vi "AutoDriver.vi"(0 "NXT In":T4, 1 "Motors":cluster{"TetrixDCMotor":T1, "TetrixDCMotor":T1}, 2 "Direction":T3=enum."Forward", 3 "Speed":T2, 5 "Time (1 sec)":sgl=1.0) -> (6 "NXT Out":T4)   [LabVIEW 2012]
uses:
  <vilib>/NXT/Subs/LVHSConnector.ctl
  <vilib>/NXT/LegoClasses/BrickReference/BrickReference.lvclass
  AutoDriverControl.ctl
  FTC 2012 - 2013/Controls/SpeedControl.ctl
  <vilib>/NXT/Hardware/Plugins/Tetrix DC Motor/TetrixDCMotorAddress.ctl
  <vilib>/NXT/Dual Mode Library/Waits/Wait_Num.vi
  <vilib>/NXT/NXTIO Xnodes/NXTIONodeSubVIs/TETRIX IO Move DC Motors.vi
  <vilib>/NXT/NXTIO Xnodes/NXTIONodeSubVIs/TETRIX IO Stop DC Motors.vi
  <vilib>/NXT/NXTIO Xnodes/NXTIOXNode/NXTIO.xnode
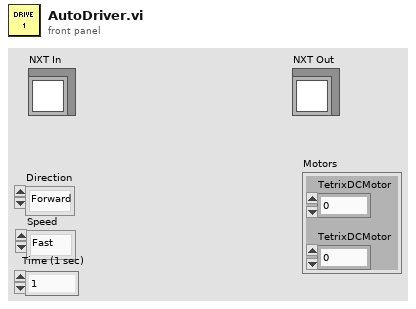
[diagram p1: front panel]
types:
  T1 = typedef "TetrixDCMotorAddress.ctl" = i16
  T2 = typedef "SpeedControl.ctl" = enum16{"Fast", "Medium", "Slow"}
  T3 = typedef "AutoDriverControl.ctl" = enum16{"Init", "Forward", "Reverse", "Left", "Right", "Brake"}
  T4 = typedef "LVHSConnector.ctl" = refnum<class "BrickReference.lvclass">
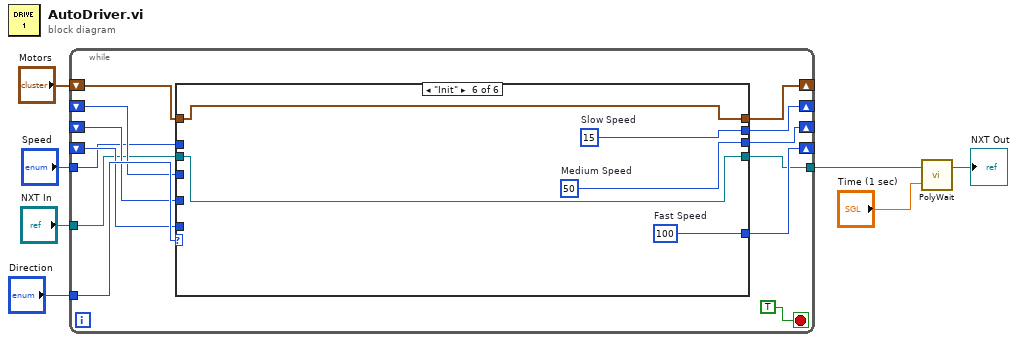
[diagram p0: block diagram]
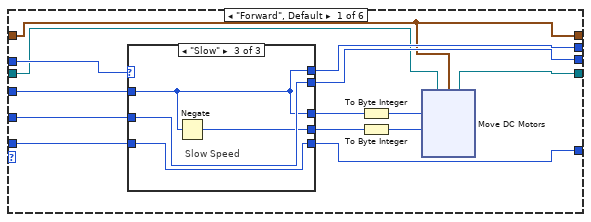
[diagram p2: hidden frame]
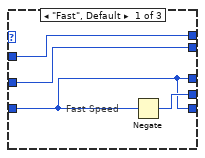
[diagram p3: hidden frame]
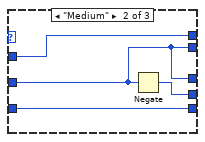
[diagram p4: hidden frame]
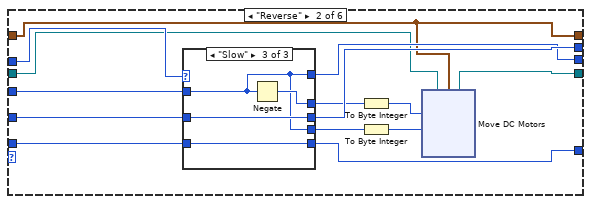
[diagram p5: hidden frame]
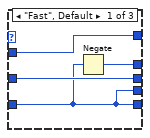
[diagram p6: hidden frame]
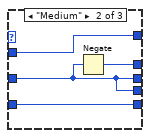
[diagram p7: hidden frame]
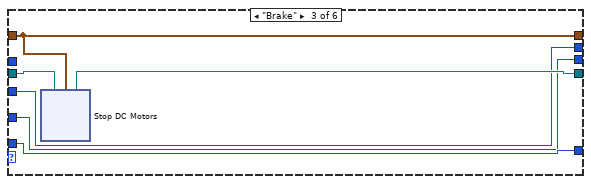
[diagram p8: hidden frame]
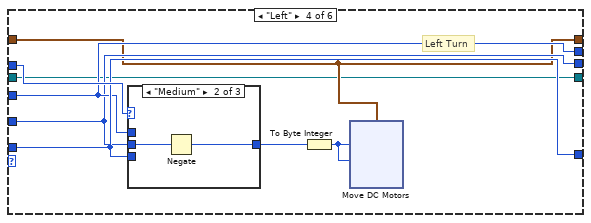
[diagram p9: hidden frame]
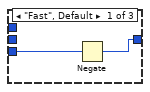
[diagram p10: hidden frame]
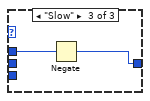
[diagram p11: hidden frame]
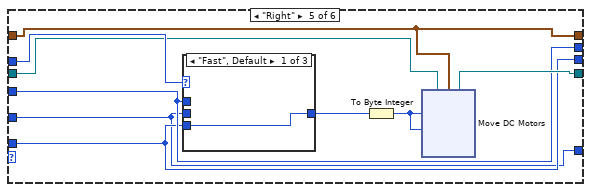
[diagram p12: hidden frame]
diagram:
  n1 = while {
    tunnel: "Direction" -> [w20]
    shift-right: [w10] -> _
    shift-left: _ -> [w17]
    shift-right: [w11] -> _
    shift-left: _ -> [w16]
    shift-right: [w18] -> _
    shift-left: _ -> [w15]
    tunnel: "NXT In" -> [w14]
    tunnel: [w13] -> w4
    tunnel: "Speed" -> [w12]
    shift-right: [w9] -> _
    shift-left: "Motors" -> [w8]
    stop <- TRUE stop-if-true
    n2 = case shown="\"Init\"" w20 {
      tunnel: [w30 w69 w94 w111 w134 w154] -> w10
      tunnel: [w31 w68 w95 w110 w133 w153] -> w11
      tunnel: [w29 w66 w96 w112 w130 w155] -> w18
      tunnel: w17 -> [w34 w63 w94 w111 w134 _]
      tunnel: w16 -> [w33 w62 w95 w110 w130 _]
      tunnel: w15 -> [w32 w70 w96 w112 w133 _]
      tunnel: w14 -> [w27 w65 w98 w108 w136 w156]
      tunnel: [w26 w64 w97 w108 w135 w156] -> w13
      tunnel: w12 -> [w28 w67 _ w113 w138 _]
      tunnel: [w21 w57 w93 w109 w137 w152] -> w9
      tunnel: w8 -> [w21 w57 w93 w109 w137 w152]
      frame "Forward", Default {
        n3 = case shown="\"Slow\"" w28 {
          tunnel: w34 -> [w47 w52 w53]
          tunnel: w33 -> [w48 w49 w55]
          tunnel: w32 -> [w45 w51 w56]
          tunnel: [w48 w49 w55] -> w31
          tunnel: [w47 w52 w53] -> w30
          tunnel: [w45 w51 w56] -> w29
          tunnel: [w46 w50 w54] -> w25
          tunnel: [w45 w49 w53] -> w23
          frame "Fast", Default {
            # "Fast Speed"
            n4 = Negate(x=w45) -> (-x=w46:i32)
          }
          frame "Medium" {
            n5 = Negate(x=w49) -> (-x=w50:i32)
          }
          frame "Slow" {
            # "Slow Speed"
            n6 = Negate(x=w53) -> (-x=w54:i32)
          }
        }
        n7 = To Byte Integer(number=w23) -> (8bit integer=w22:i8)
        n8 = To Byte Integer(number=w25) -> (8bit integer=w24:i8)
        n9 = xnode "Move DC Motors"("Power/Speed 2"=w24, "Power/Speed 1"=w22, "Motors"=w21, "NXT"=w27) -> ("NXT"=w26:T4)
      }
      frame "Reverse" {
        n10 = case shown="\"Slow\"" w67 {
          tunnel: w62 -> [w83 w85 w92]
          tunnel: w63 -> [w84 w88 w89]
          tunnel: w70 -> [w81 w87 w91]
          tunnel: [w84 w88 w89] -> w68
          tunnel: [w83 w85 w92] -> w69
          tunnel: [w82 w86 w90] -> w59
          tunnel: [w81 w87 w91] -> w66
          tunnel: [w81 w85 w89] -> w61
          frame "Fast", Default {
            n11 = Negate(x=w81) -> (-x=w82:i32)
          }
          frame "Medium" {
            n12 = Negate(x=w85) -> (-x=w86:i32)
          }
          frame "Slow" {
            n13 = Negate(x=w89) -> (-x=w90:i32)
          }
        }
        n14 = To Byte Integer(number=w59) -> (8bit integer=w58:i8)
        n15 = To Byte Integer(number=w61) -> (8bit integer=w60:i8)
        n16 = xnode "Move DC Motors"("Power/Speed 2"=w60, "Power/Speed 1"=w58, "Motors"=w57, "NXT"=w65) -> ("NXT"=w64:T4)
      }
      frame "Brake" {
        n17 = xnode "Stop DC Motors"("Motors"=w93, "NXT"=w98) -> ("NXT"=w97:T4)
      }
      frame "Left" {
        # "Left Turn"
        n18 = case shown="\"Medium\"" w113 {
          tunnel: w112 -> [w125 _ _]
          tunnel: [w124 w126 w128] -> w106
          tunnel: w110 -> [_ w127 _]
          tunnel: w111 -> [_ _ w129]
          frame "Fast", Default {
            n19 = Negate(x=w125) -> (-x=w124:i32)
          }
          frame "Medium" {
            n20 = Negate(x=w127) -> (-x=w126:i32)
          }
          frame "Slow" {
            n21 = Negate(x=w129) -> (-x=w128:i32)
          }
        }
        n22 = To Byte Integer(number=w106) -> (8bit integer=w107:i8)
        n23 = xnode "Move DC Motors"("Power/Speed 2"=w107, "Power/Speed 1"=w107, "Motors"=w109) -> ()  [unwired: 1 in, 1 out]
      }
      frame "Right" {
        n24 = case shown="\"Fast\", Default" w138 {
          tunnel: [w149 w150 w151] -> w132
          tunnel: w130 -> [_ w150 _]
          tunnel: w134 -> [_ _ w151]
          tunnel: w133 -> [w149 _ _]
          frame "Fast", Default {
          }
          frame "Medium" {
          }
          frame "Slow" {
          }
        }
        n25 = To Byte Integer(number=w132) -> (8bit integer=w131:i8)
        n26 = xnode "Move DC Motors"("Power/Speed 2"=w131, "Power/Speed 1"=w131, "Motors"=w137, "NXT"=w136) -> ("NXT"=w135:T4)
      }
      frame "Init" {
        w153 = 50  # Medium Speed
        w154 = 15  # Slow Speed
        w155 = 100  # Fast Speed
      }
    }
  }
  n27 = call-poly <vilib>:"PolyWait.vi"("Time (1 sec)"="Time (1 sec)", "NXT"=w4) -> ("NXT"=→"NXT Out":T4)  [unwired: 2 in]
